vi "2_8.vi"() -> ()   [LabVIEW 2015]
panel:
  out "Element":dbl
  in  "Index":i32
  out "initialized array":dbl[](array[numeric])
  out "Threshold Index":dbl
  out "Rotated Array":dbl[](array[numeric])
  out "Reverse Array":dbl[](array[numeric])
  out "Sort Array":dbl[](array[numeric])
  out "Min index(es)":i32
  out "Min":dbl
  out "Max index(es)":i32
  out "Max":dbl
  out "Array Subset":dbl[](array[numeric])
  out "Insert Array":dbl[](array[numeric])
  out "Match Index":i32
  out "Size":i32
  out "Build Array":dbl[](array[numeric])
  in  "Numeric":dbl
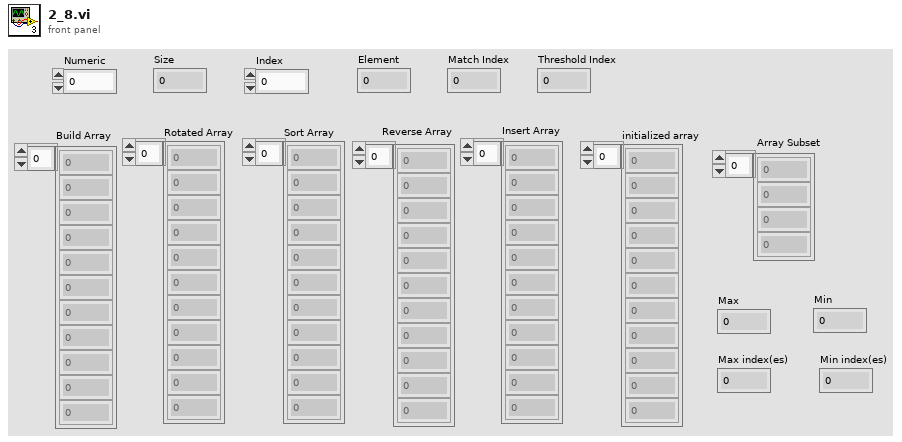
[diagram p1: front panel]
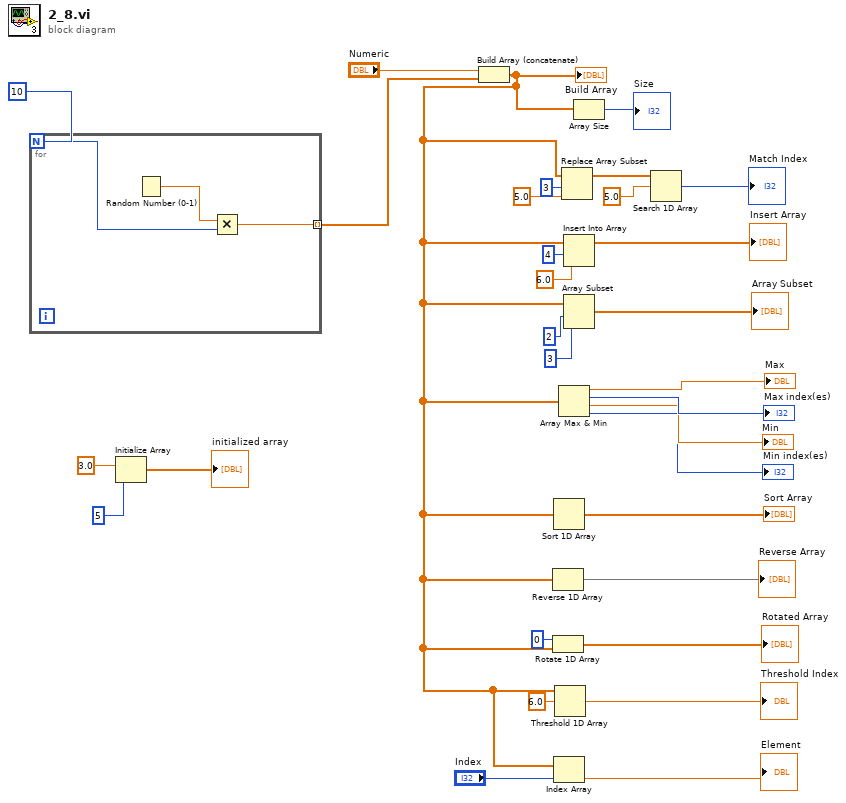
[diagram p0: block diagram]
diagram:
  n1 = for {
    N: 10 -> [w33]
    tunnel: [w32] -> w5 mode=indexing
    n2 = Random Number (0-1)() -> (number: 0 to 1=w34:dbl)
    n3 = Multiply(x=w34, y=w33) -> (x*y=w32:dbl)
  }
  n4 = Initialize Array(3.0 ("element"), 5 ("dimension size")) -> (→"initialized array":dbl[])
  n5 = Build Array (concatenate)("Numeric", w5) -> (w2:dbl[])
  "Build Array" <- w2
  n6 = Reverse 1D Array(array=w2) -> (reversed array=→"Reverse Array":dbl[])
  n7 = Rotate 1D Array(1:w2, 2:0 ("n")) -> (0:→"Rotated Array":dbl[])
  n8 = Sort 1D Array(array=w2) -> (sorted array=→"Sort Array":dbl[])
  n9 = Index Array(array=w2, index="Index") -> (element=→"Element":dbl)
  n10 = Threshold 1D Array(2:6.0 ("threshold y"), 3:w2) -> (0:→"Threshold Index":dbl)  [unwired: 1 in]
  n11 = Array Max & Min(array=w2) -> (max value=→"Max":dbl, max index (indices)=→"Max index(es)":i32, min value=→"Min":dbl, min index (indices)=→"Min index(es)":i32)
  n12 = Replace Array Subset(array=w2, new element=5.0 ("new element/subarray"), index=3) -> (w25:dbl[])
  n13 = Insert Into Array(array=w2, index=4, new element=6.0 ("new element/subarray")) -> (→"Insert Array":dbl[])
  n14 = Array Subset(array=w2, index=2, length=3) -> (→"Array Subset":dbl[])
  n15 = Array Size(array=w2) -> (size(s)=→"Size":i32)
  n16 = Search 1D Array(1D array=w25, element=5.0) -> (index of element=→"Match Index":i32)  [unwired: 1 in]
